vi "HFRR ADV v017 new software.vi"() -> ()   [LabVIEW 2025] (continued)
            n3480 = property on="File Path" class="Path"("Caption.Text"=w4485) -> ()  [unwired: 2 in, 2 out]
            n3481 = property on="SrvM CP" class="Bool (strict)"("Boolean Text.Text"=w4484) -> ()  [unwired: 2 in, 2 out]
            n3482 = local read "S 71"() -> (w4479:string)
            n3483 = local read "S 86"() -> (w4481:string)
            n3484 = local read "S 85"() -> (w4482:string)
            n3485 = local read "S 87"() -> (w4480:string)
            n3486 = local read "S 84"() -> (w4483:string)
            n3487 = local read "S 103"() -> (w4468:string)
            n3488 = local read "S 104"() -> (w4467:string)
            n3489 = property on="ENTER THE NEW PASSWORD" class="Str"("Caption.Text"=w4480) -> ()  [unwired: 2 in, 2 out]
            n3490 = property on="Password" class="Str"("Caption.Text"=w4482) -> ()  [unwired: 2 in, 2 out]
            n3491 = property on="ENTER CURRENT PASSWORD" class="Str"("Caption.Text"=w4481) -> ()  [unwired: 2 in, 2 out]
            n3492 = property on="EDIT" class="Bool (strict)"("Boolean Text.Text"=w4479) -> ()  [unwired: 2 in, 2 out]
            n3493 = property on="SAVE" class="Bool (strict)"("Boolean Text.Text"=w4483) -> ()  [unwired: 2 in, 2 out]
            n3494 = Build Array(w4468, w4467) -> (w4466:string[])
            n3495 = property on="Heater Button" class="Bool (strict)"("Strings [4]"=w4466) -> ()  [unwired: 2 in, 2 out]
            n3496 = property on="CH-HUMIDITY WET" class="DigNum (strict)"("Caption.Size to Text?"=w4469) -> ()  [unwired: 2 in, 2 out]
            n3497 = property on="CH-HUMIDITY DRY" class="DigNum (strict)"("Caption.Size to Text?"=w4469) -> ()  [unwired: 2 in, 2 out]
            n3498 = property on="CH-POWER -" class="DigNum (strict)"("Caption.Size to Text?"=w4469) -> ()  [unwired: 2 in, 2 out]
            n3499 = property on="CH-HEATER" class="DigNum (strict)"("Caption.Size to Text?"=w4469) -> ()  [unwired: 2 in, 2 out]
            n3500 = property on="CH-POWER +" class="DigNum (strict)"("Caption.Size to Text?"=w4469) -> ()  [unwired: 2 in, 2 out]
            n3501 = local read "S 92"() -> (w4478:string)
            n3502 = local read "S 93"() -> (w4477:string)
            n3503 = local read "S 105"() -> (w4464:string)
            n3504 = local read "S 106"() -> (w4463:string)
            n3505 = Build Array(w4478, w4477) -> ()  [unwired: 1 out]
            n3506 = Build Array(w4464, w4463) -> (w4465:string[])
            n3507 = local read "S 95"() -> (w4475:string)
            n3508 = local read "S 94"() -> (w4476:string)
            n3509 = local read "bs"() -> (w4491:string)
            n3510 = local read "as"() -> (w4492:string)
            n3511 = property on="Humidity" class="Bool (strict)"("Strings [4]"=w4465) -> ()  [unwired: 2 in, 2 out]
            n3512 = Concatenate Strings(w4491, "\r", w4492) -> ()  [unwired: 1 out]
            n3513 = property on="STROKE GAIN :" class="DigNum (strict)"("Caption.Text"=w4475) -> ()  [unwired: 2 in, 2 out]
            n3514 = property on="DISPLACEMENT :" class="DigNum (strict)"("Caption.Text"=w4476) -> ()  [unwired: 2 in, 2 out]
            n3515 = property on="Rh After" class="DigNum (strict)"("Caption.Size to Text?"=TRUE ("Caption.Size to Text")) -> ()  [unwired: 2 in, 2 out]
            n3516 = local read "S 48"() -> (w4515:string)
            n3517 = local read "S 50"() -> (w4513:string)
            n3518 = local read "S 51"() -> (w4512:string)
            n3519 = local read "S 49"() -> (w4514:string)
            n3520 = local read "S 52"() -> (w4511:string)
            n3521 = local read "as"() -> (w4496:string)
            n3522 = local read "bs"() -> (w4497:string)
            n3523 = local read "S 56"() -> (w4510:string)
            n3524 = local read "S 57"() -> (w4509:string)
            n3525 = local read "S 58"() -> (w4508:string)
            n3526 = local read "S 59"() -> (w4507:string)
            n3527 = property on="OPEN" class="Bool (strict)"("Boolean Text.Text"=w4511) -> ()  [unwired: 2 in, 2 out]
            n3528 = property on="OPEN 1" class="Bool (strict)"("Boolean Text.Text"=w4515) -> ()  [unwired: 2 in, 2 out]
            n3529 = property on="OPEN 2" class="Bool (strict)"("Boolean Text.Text"=w4514) -> ()  [unwired: 2 in, 2 out]
            n3530 = property on="OPEN 3" class="Bool (strict)"("Boolean Text.Text"=w4513) -> ()  [unwired: 2 in, 2 out]
            n3531 = property on="OPEN 4" class="Bool (strict)"("Boolean Text.Text"=w4512) -> ()  [unwired: 2 in, 2 out]
            n3532 = Concatenate Strings(w4497, "\r", w4496) -> ()  [unwired: 1 out]
            n3533 = local read "S 102"() -> (w4470:string)
            n3534 = property on="КОФ1" class="DigNum (strict)"("Caption.Text"=w4510) -> ()  [unwired: 2 in, 2 out]
            n3535 = local read "S 98"() -> (w4474:string)
            n3536 = local read "S 99"() -> (w4473:string)
            n3537 = local read "S 100"() -> (w4472:string)
            n3538 = local read "S 101"() -> (w4471:string)
            n3539 = property on="КОФ2" class="DigNum (strict)"("Caption.Text"=w4509) -> ()  [unwired: 2 in, 2 out]
            n3540 = property on="КОФ3" class="DigNum (strict)"("Caption.Text"=w4508) -> ()  [unwired: 2 in, 2 out]
            n3541 = property on="КОФ4" class="DigNum (strict)"("Caption.Text"=w4507) -> ()  [unwired: 2 in, 2 out]
            n3542 = local read "bs"() -> (w4495:string)
            n3543 = local read "as"() -> (w4494:string)
            n3544 = property on="CH-POWER +" class="DigNum (strict)"("Caption.Text"=w4474) -> ()  [unwired: 2 in, 2 out]
            n3545 = property on="CH-POWER -" class="DigNum (strict)"("Caption.Text"=w4473) -> ()  [unwired: 2 in, 2 out]
            n3546 = property on="CH-HEATER" class="DigNum (strict)"("Caption.Text"=w4472) -> ()  [unwired: 2 in, 2 out]
            n3547 = property on="CH-HUMIDITY DRY" class="DigNum (strict)"("Caption.Text"=w4471) -> ()  [unwired: 2 in, 2 out]
            n3548 = property on="CH-HUMIDITY WET" class="DigNum (strict)"("Caption.Text"=w4470) -> ()  [unwired: 2 in, 2 out]
            n3549 = local read "S 60"() -> (w4506:string)
            n3550 = local read "S 54"() -> (w4516:string)
            n3551 = Concatenate Strings(w4495, "\r", w4494) -> ()  [unwired: 1 out]
            n3552 = Concatenate Strings(w4516, w4506) -> ()  [unwired: 1 out]
            n3553 = local read "S 77"() -> (→"String 43":string)
            n3554 = local read "S 76"() -> (w4489:string)
            n3555 = local read "S 78"() -> (w4488:string)
            n3556 = local read "S 71"() -> (w4500:string)
            n3557 = local read "S 66"() -> (w4505:string)
            n3558 = local read "S 67"() -> (w4504:string)
            n3559 = local read "S 68"() -> (w4503:string)
            n3560 = local read "S 69"() -> (w4502:string)
            n3561 = local read "S 70"() -> (w4501:string)
            n3562 = property on="AIR TEMP" class="DigNum (strict)"("Caption.Text"=w4488) -> ()  [unwired: 2 in, 2 out]
            n3563 = property on="Set Strk" class="DigNum (strict)"("Caption.Text"=w4489) -> ()  [unwired: 2 in, 2 out]
            n3564 = property on="FRIC. FORCE :" class="DigNum (strict)"("Caption.Text"=w4505) -> ()  [unwired: 2 in, 2 out]
            n3565 = property on="TEMPERATURE :" class="DigNum (strict)"("Caption.Text"=w4504) -> ()  [unwired: 2 in, 2 out]
            n3566 = property on="SPEED OUT:" class="DigNum (strict)"("Caption.Text"=w4503) -> ()  [unwired: 2 in, 2 out]
            n3567 = property on="AIR TEMPERATURE :" class="DigNum (strict)"("Caption.Text"=w4502) -> ()  [unwired: 2 in, 2 out]
            n3568 = property on="HUMIDITY:" class="DigNum (strict)"("Caption.Text"=w4501) -> ()  [unwired: 2 in, 2 out]
            n3569 = property on="EDIT" class="Bool (strict)"("Boolean Text.Text"=w4500) -> ()  [unwired: 2 in, 2 out]
            n3570 = local read "S 79"() -> (w4487:string)
          }
          frame #2 {
          }
        }
        n3571 = local write "Lan flag"(10.0 ("Lan flag")) -> ()
      }
      frame Enabled {
      }
    }
    n3572 = Wait (ms)(milliseconds to wait=u32 2000) -> ()  [unwired: 1 out]
    n3573 = local read "Quit"() -> (w4290:bool)
  }
  n3574 = while {
    shift-right: [w4522] -> _
    shift-left: _ -> [w4523]
    shift-right: [w4520] -> _
    shift-left: T18 {"Read Heave and Surge"="", "Bytes at Heave Port"=0.0, "Heave and Surge COM Port:"="COM9", "Com Port 2"="COM7", "Residual Due"="", "Heave COM Status 2"=TRUE, "Heave COM Status"=TRUE, "Port 2"=TRUE, "Sway PPR"=6400.0, "Surge PPR"=6400.0, "Heave PPR"=6400.0, "Sway Pitch"=2.0, "Surge Pitch"=3.0, "Heave Pitch"=4.0, "Sway Pulses/mm"=320.0, "Surge Pulses/mm"=1600.0, "Heave Pulses/mm"=1600.0, "inner loop"=0.0, "Read Heave and Surge 2"="", "String 36"="", "Write S"=FALSE, "WriteCC1"=[""], "Heave COM Loop"=0, "LastCom"="", "EXIT"=FALSE, "Error Heave"={"status"=TRUE, "code"=-1073807343, "source"=""}} -> [w4519]
    shift-right: [w4517] -> _
    shift-left: _ -> [w4518]
    stop <- w4521 stop-if-true
    n3575 = case shown="\"init\"" w4518 {
      tunnel: w4523 -> [w4537 w4552 w4613 w4615]
      tunnel: [w4532 w4561 w4613 w4615] -> w4522
      tunnel: [_ _ TRUE _] -> w4521
      tunnel: [w4528 w4558 w4611 w4614] -> w4520
      tunnel: w4519 -> [w4534 w4551 w4611 w4614]
      tunnel: [enum16{"init", "MAIN", "Panel Close"}."MAIN" w4545 _ _] -> w4517
      frame "init" {
        n3576 = local read "Com Port 1"() -> (w4524:refnum<visa-resource-name>)
        n3577 = Bundle By Name(cluster=w4534, "Com Port 2"=w4524) -> (w4533:T18)
        n3578 = call "Instrument fgv.vi"("Enum"=T31."INIT", "error in (no error) 2"=w4537, "INPUT"=w4533) -> ("error"=w4535:errorcluster, "output"=w4531:T18)  [unwired: 6 in, 1 out]
        n3579 = case shown="Error" w4535 {
          selector: w4535 -> [w4539 _]
          tunnel: [w4539 w4543] -> w4532
          tunnel: w4531 -> [w4538 w4541]
          tunnel: [w4538 w4540] -> w4529
          frame No Error {
          }
          frame Error {
            n3580 = call "Instrument fgv.vi"("Enum"=T31."ERROR INIT", "INPUT"=w4541) -> ("error"=w4544:errorcluster, "output"=w4540:T18)  [unwired: 7 in, 1 out]
            n3581 = call <vilib>:"Clear Errors.vi"("error in (no error)"=w4544) -> ("error out"=w4543:errorcluster)  [unwired: 5 in, 1 out]
          }
        }
        n3582 = local read "LastCom 2"() -> (w4527:string)
        n3583 = Unbundle By Name(w4529) -> ("Heave COM Status 2"=→"COM Status 2" →"Instrument Status 2":bool, "Error Heave"=→"Error  2":errorcluster)  [unwired: 1 out]
        n3584 = Bundle By Name(cluster=w4529, "LastCom"=w4527) -> (w4528:T18)
      }
      frame "MAIN" {
        n3585 = Unbundle By Name(w4551) -> ("Com Port 2"=w4563:refnum<visa-resource-name>)
        n3586 = local write "Com Port 5"(w4563) -> ()
        n3587 = local read item#-1() -> (w4549)
        n3588 = Bundle By Name(cluster=w4551, "Heave and Surge COM Port:"=w4549) -> (w4550:T18)
        n3589 = Equal?(x=w4563, y=w4549) -> (x = y?=w4562:bool)
        n3590 = case shown="True" w4562 {
          tunnel: [w4567 w4584] -> w4561
          tunnel: w4552 -> [w4568 w4590]
          tunnel: w4550 -> [w4566 w4588]
          tunnel: [w4565 w4583] -> w4558
          frame False {
            n3591 = call <vilib>:"Clear Errors.vi"("error in (no error)"=w4568) -> ("error out"=w4564:errorcluster)  [unwired: 5 in, 1 out]
            n3592 = call "Instrument fgv.vi"("Enum"=T31."ERROR INIT", "error in (no error) 2"=w4564, "INPUT"=w4566) -> ("error"=w4570:errorcluster, "output"=w4565:T18)  [unwired: 6 in, 1 out]
            n3593 = call <vilib>:"Clear Errors.vi"("error in (no error)"=w4570) -> ("error out"=w4567:errorcluster)  [unwired: 5 in, 1 out]
          }
          frame True {
            n3594 = call "Instrument fgv.vi"("Enum"=T31."READ", "error in (no error) 2"=w4590, "INPUT"=w4588) -> ("error"=w4589:errorcluster, "output"=w4580:T18)  [unwired: 6 in, 1 out]
            n3595 = Bundle By Name(cluster=w4580, "String 36"="String 15") -> (w4579:T18)
            n3596 = case shown="True" "Write S 2" {
              selector: "Write S 2" -> [_ w4610]
              tunnel: w4589 -> [w4603 w4609]
              tunnel: [w4603 w4608] -> w4576
              tunnel: w4579 -> [w4602 w4605]
              tunnel: [w4602 w4604] -> w4575
              frame False {
              }
              frame True {
                n3597 = Not(x=w4610) -> (.not. x?=w4606:bool)
                n3598 = local write "Write S 2"(w4606) -> ()
                n3599 = call "Instrument fgv.vi"("Enum"=T31."MANUAL WRITE", "error in (no error) 2"=w4609, "INPUT"=w4605) -> ("error"=w4608:errorcluster, "output"=w4604:T18)  [unwired: 6 in, 1 out]
              }
            }
            n3600 = Array Size(array="WriteHumidity 2") -> (size(s)=w4573:i32)
            n3601 = Greater Than 0?(x=w4573) -> (x > 0?=w4571:bool)
            n3602 = call "Instrument fgv.vi"("Enum"=T31."WRITE", "error in (no error) 2"=w4576, "WriteCC1"="WriteHumidity 2", "INPUT"=w4575) -> ("error"=w4586:errorcluster, "WriteCC1 2"=w4574:string[], "output"=w4585:T18)  [unwired: 5 in]
            n3603 = case shown="Error" w4586 {
              selector: w4586 -> [w4593 w4596]
              tunnel: w4585 -> [w4594 w4601]
              tunnel: [w4594 w4600] -> w4583
              tunnel: [w4593 w4598] -> w4584
              frame No Error {
              }
              frame Error {
                n3604 = call <vilib>:"Clear Errors.vi"("error in (no error)"=w4596) -> ("error out"=w4595:errorcluster)  [unwired: 5 in, 1 out]
                n3605 = call "Instrument fgv.vi"("Enum"=T31."ERROR INIT", "error in (no error) 2"=w4595, "INPUT"=w4601) -> ("error"=w4599:errorcluster, "output"=w4600:T18)  [unwired: 6 in, 1 out]
                n3606 = call <vilib>:"Clear Errors.vi"("error in (no error)"=w4599) -> ("error out"=w4598:errorcluster)  [unwired: 5 in, 1 out]
              }
            }
            n3607 = case shown="True" w4571 {
              tunnel: w4574 -> [_ w4592]
              frame False {
              }
              frame True {
                n3608 = local write "WriteHumidity 2"(w4592) -> ()
              }
            }
            n3609 = Unbundle By Name(w4583) -> ("LastCom"=→"LastCom 2":string, "Read Heave and Surge"=→"Read Humidity 2":string)
          }
        }
        n3610 = Unbundle By Name(w4558) -> ("Heave COM Status 2"=w4560:bool, "Heave COM Status"=w4559:bool, "Error Heave"=w4556:errorcluster, "Bytes at Heave Port"=→"Bytes at Humidity Port  2":dbl)
        n3611 = Unbundle By Name(w4556) -> ("status"=→"Humidity Port 2":bool)
        n3612 = Not(x=w4559) -> (.not. x?=w4553:bool)
        n3613 = local write "Error  2"(w4556) -> ()
        n3614 = Not(x=w4560) -> (.not. x?=w4554:bool)
        n3615 = local write "Instrument Status 2"(w4553) -> ()
        n3616 = local write "COM Status 2"(w4554) -> ()
        n3617 = local read "Quit"() -> (w4546:bool)
        n3618 = Select(t=enum16{"init", "MAIN", "Panel Close"}."Panel Close", s=w4546, f=enum16{"init", "MAIN", "Panel Close"}."MAIN") -> (s? t:f=w4545:enum16{"init", "MAIN", "Panel Close"})
      }
      frame "Panel Close" {
      }
      frame Default {
      }
    }
  }
  n3619 = disable-structure shown="Disabled" {
    frame Disabled {
      n3620 = while {
        tunnel: [w4617] -> _
        i -> [w4617]
        stop <- w4616 continue-if-true
        n3621 = Wait (ms)(milliseconds to wait=u32 50) -> ()  [unwired: 1 out]
        n3622 = stacked-sequence {
          frame #0 {
            # "Controls Text color"
            # "Controls BG color"
            n3623 = property on="FILE" class="Str"("Text.Text Colors:Text Color"="SC  Text") -> ()  [unwired: 2 in, 2 out]
            n3624 = property on="Fuel Discription :" class="Str"("Text.Text Colors:Text Color"="SC  Text") -> ()  [unwired: 2 in, 2 out]
            n3625 = property on="tested by" class="Str"("Text.Text Colors:Text Color"="SC  Text") -> ()  [unwired: 2 in, 2 out]
            n3626 = property on="Remarks :" class="Str"("Text.Text Colors:Text Color"="SC  Text") -> ()  [unwired: 2 in, 2 out]
            n3627 = property class="DigNum (strict)"("Numeric Text.Text Colors:BG Color"="NC BG") -> ()  [unwired: 2 in, 2 out]
            n3628 = property class="DigNum (strict)"("Numeric Text.Text Colors:BG Color"="NC BG") -> ()  [unwired: 2 in, 2 out]
            n3629 = property class="DigNum (strict)"("Numeric Text.Text Colors:BG Color"="NC BG") -> ()  [unwired: 2 in, 2 out]
            n3630 = property class="DigNum (strict)"("Numeric Text.Text Colors:BG Color"="NC BG") -> ()  [unwired: 2 in, 2 out]
            n3631 = property class="DigNum (strict)"("Numeric Text.Text Colors:BG Color"="NC BG") -> ()  [unwired: 2 in, 2 out]
            n3632 = property class="DigNum (strict)"("Numeric Text.Text Colors:BG Color"="NC BG") -> ()  [unwired: 2 in, 2 out]
            n3633 = property class="DigNum (strict)"("Numeric Text.Text Colors:BG Color"="NC BG") -> ()  [unwired: 2 in, 2 out]
            n3634 = property class="DigNum (strict)"("Numeric Text.Text Colors:BG Color"="NC BG") -> ()  [unwired: 2 in, 2 out]
            n3635 = property class="DigNum (strict)"("Numeric Text.Text Colors:BG Color"="NC BG") -> ()  [unwired: 2 in, 2 out]
            n3636 = property class="DigNum (strict)"("Numeric Text.Text Colors:BG Color"="NC BG") -> ()  [unwired: 2 in, 2 out]
            n3637 = property class="DigNum (strict)"("Numeric Text.Text Colors:BG Color"="NC BG") -> ()  [unwired: 2 in, 2 out]
            n3638 = property class="DigNum (strict)"("Numeric Text.Text Colors:BG Color"="NC BG") -> ()  [unwired: 2 in, 2 out]
            n3639 = property on="FILE" class="Str"("Text.Text Colors:BG Color"="SC BG 3") -> ()  [unwired: 2 in, 2 out]
            n3640 = property on="Fuel Discription :" class="Str"("Text.Text Colors:BG Color"="SC BG 3") -> ()  [unwired: 2 in, 2 out]
            n3641 = property on="tested by" class="Str"("Text.Text Colors:BG Color"="SC BG 3") -> ()  [unwired: 2 in, 2 out]
            n3642 = property on="Remarks :" class="Str"("Text.Text Colors:BG Color"="SC BG 3") -> ()  [unwired: 2 in, 2 out]
            n3643 = property class="DigNum (strict)"("Numeric Text.Text Colors:Text Color"="NC Text") -> ()  [unwired: 2 in, 2 out]
            n3644 = property class="DigNum (strict)"("Numeric Text.Text Colors:Text Color"="NC Text") -> ()  [unwired: 2 in, 2 out]
            n3645 = property class="DigNum (strict)"("Numeric Text.Text Colors:Text Color"="NC Text") -> ()  [unwired: 2 in, 2 out]
            n3646 = property class="DigNum (strict)"("Numeric Text.Text Colors:Text Color"="NC Text") -> ()  [unwired: 2 in, 2 out]
            n3647 = property class="DigNum (strict)"("Numeric Text.Text Colors:Text Color"="NC Text") -> ()  [unwired: 2 in, 2 out]
            n3648 = property class="DigNum (strict)"("Numeric Text.Text Colors:Text Color"="NC Text") -> ()  [unwired: 2 in, 2 out]
            n3649 = property class="DigNum (strict)"("Numeric Text.Text Colors:Text Color"="NC Text") -> ()  [unwired: 2 in, 2 out]
            n3650 = property class="DigNum (strict)"("Numeric Text.Text Colors:Text Color"="NC Text") -> ()  [unwired: 2 in, 2 out]
            n3651 = property class="DigNum (strict)"("Numeric Text.Text Colors:Text Color"="NC Text") -> ()  [unwired: 2 in, 2 out]
            n3652 = property class="DigNum (strict)"("Numeric Text.Text Colors:Text Color"="NC Text") -> ()  [unwired: 2 in, 2 out]
            n3653 = property class="DigNum (strict)"("Numeric Text.Text Colors:Text Color"="NC Text") -> ()  [unwired: 2 in, 2 out]
            n3654 = property class="DigNum (strict)"("Numeric Text.Text Colors:Text Color"="NC Text") -> ()  [unwired: 2 in, 2 out]
            n3655 = property class="DigNum (strict)"("Numeric Text.Text Colors:Text Color"="NI Text  2") -> ()  [unwired: 2 in, 2 out]
            n3656 = property class="DigNum (strict)"("Numeric Text.Text Colors:Text Color"="NI Text  2") -> ()  [unwired: 2 in, 2 out]
            n3657 = property class="DigNum (strict)"("Numeric Text.Text Colors:Text Color"="NI Text  2") -> ()  [unwired: 2 in, 2 out]
            n3658 = property class="DigNum (strict)"("Numeric Text.Text Colors:Text Color"="NI Text  2") -> ()  [unwired: 2 in, 2 out]
            n3659 = property class="DigNum (strict)"("Numeric Text.Text Colors:Text Color"="NI Text  2") -> ()  [unwired: 2 in, 2 out]
            n3660 = property class="DigNum (strict)"("Numeric Text.Text Colors:Text Color"="NI Text  2") -> ()  [unwired: 2 in, 2 out]
            n3661 = property class="DigNum (strict)"("Numeric Text.Text Colors:Text Color"="NI Text  2") -> ()  [unwired: 2 in, 2 out]
            n3662 = property class="DigNum (strict)"("Numeric Text.Text Colors:Text Color"="NI Text  2") -> ()  [unwired: 2 in, 2 out]
            n3663 = property class="DigNum (strict)"("Numeric Text.Text Colors:Text Color"="NI Text  2") -> ()  [unwired: 2 in, 2 out]
            n3664 = property class="DigNum (strict)"("Numeric Text.Text Colors:Text Color"="NI Text  2") -> ()  [unwired: 2 in, 2 out]
            n3665 = property class="DigNum (strict)"("Numeric Text.Text Colors:Text Color"="NI Text  2") -> ()  [unwired: 2 in, 2 out]
            n3666 = property class="DigNum (strict)"("Numeric Text.Text Colors:Text Color"="NI Text  2") -> ()  [unwired: 2 in, 2 out]
            n3667 = property class="DigNum (strict)"("Numeric Text.Text Colors:Text Color"="NI Text  2") -> ()  [unwired: 2 in, 2 out]
            n3668 = property class="DigNum (strict)"("Numeric Text.Text Colors:Text Color"="NI Text  2") -> ()  [unwired: 2 in, 2 out]
            n3669 = property class="DigNum (strict)"("Numeric Text.Text Colors:Text Color"="NI Text  2") -> ()  [unwired: 2 in, 2 out]
            n3670 = property on="Coefficient Of Friction" class="XYGraph (strict)"("Plot Area:Colors:FG Color"="GFG  2", "Plot Area:Colors:BG Color"="GBG   2") -> ()  [unwired: 2 in, 2 out]
            n3671 = property on="Humidity ( %RH )" class="XYGraph (strict)"("Plot Area:Colors:FG Color"="GFG  2", "Plot Area:Colors:BG Color"="GBG   2") -> ()  [unwired: 2 in, 2 out]
            n3672 = property on="Air Temperature  ( °C )" class="XYGraph (strict)"("Plot Area:Colors:FG Color"="GFG  2", "Plot Area:Colors:BG Color"="GBG   2") -> ()  [unwired: 2 in, 2 out]
            n3673 = property on="Sample Temperature ( °C )" class="XYGraph (strict)"("Plot Area:Colors:FG Color"="GFG  2", "Plot Area:Colors:BG Color"="GBG   2") -> ()  [unwired: 2 in, 2 out]
            n3674 = property class="DigNum (strict)"("Numeric Text.Text Colors:BG Color"="NI BG 2") -> ()  [unwired: 2 in, 2 out]
            n3675 = property class="DigNum (strict)"("Numeric Text.Text Colors:BG Color"="NI BG 2") -> ()  [unwired: 2 in, 2 out]
            n3676 = property class="DigNum (strict)"("Numeric Text.Text Colors:BG Color"="NI BG 2") -> ()  [unwired: 2 in, 2 out]
            n3677 = property class="DigNum (strict)"("Numeric Text.Text Colors:BG Color"="NI BG 2") -> ()  [unwired: 2 in, 2 out]
            n3678 = property class="DigNum (strict)"("Numeric Text.Text Colors:BG Color"="NI BG 2") -> ()  [unwired: 2 in, 2 out]
            n3679 = property class="DigNum (strict)"("Numeric Text.Text Colors:BG Color"="NI BG 2") -> ()  [unwired: 2 in, 2 out]
            n3680 = property class="DigNum (strict)"("Numeric Text.Text Colors:BG Color"="NI BG 2") -> ()  [unwired: 2 in, 2 out]
            n3681 = property class="DigNum (strict)"("Numeric Text.Text Colors:BG Color"="NI BG 2") -> ()  [unwired: 2 in, 2 out]
            n3682 = property class="DigNum (strict)"("Numeric Text.Text Colors:BG Color"="NI BG 2") -> ()  [unwired: 2 in, 2 out]
            n3683 = property class="DigNum (strict)"("Numeric Text.Text Colors:BG Color"="NI BG 2") -> ()  [unwired: 2 in, 2 out]
            n3684 = property class="DigNum (strict)"("Numeric Text.Text Colors:BG Color"="NI BG 2") -> ()  [unwired: 2 in, 2 out]
            n3685 = property class="DigNum (strict)"("Numeric Text.Text Colors:BG Color"="NI BG 2") -> ()  [unwired: 2 in, 2 out]
            n3686 = property class="DigNum (strict)"("Numeric Text.Text Colors:BG Color"="NI BG 2") -> ()  [unwired: 2 in, 2 out]
            n3687 = property class="DigNum (strict)"("Numeric Text.Text Colors:BG Color"="NI BG 2") -> ()  [unwired: 2 in, 2 out]
            n3688 = property class="DigNum (strict)"("Numeric Text.Text Colors:BG Color"="NI BG 2") -> ()  [unwired: 2 in, 2 out]
            n3689 = property class="Bool"("Colors [4]"="Boolean BC T & BG") -> ()  [unwired: 2 in, 2 out]
            n3690 = property on="Save & Continue" class="Bool (strict)"("Colors [4]"="Boolean BC T & BG") -> ()  [unwired: 2 in, 2 out]
            n3691 = property on="Heater Button" class="Bool (strict)"("Colors [4]"="Boolean BC T & BG") -> ()  [unwired: 2 in, 2 out]
            n3692 = property class="Bool"("Colors [4]"="Boolean BC T & BG") -> ()  [unwired: 2 in, 2 out]
            n3693 = property on="Humidity" class="Bool (strict)"("Colors [4]"="Boolean BC T & BG") -> ()  [unwired: 2 in, 2 out]
            n3694 = property class="Bool (strict)"("Colors [4]"="Boolean BC T & BG") -> ()  [unwired: 2 in, 2 out]
            n3695 = property on="RUN" class="Bool (strict)"("Colors [4]"="Boolean BC T & BG") -> ()  [unwired: 2 in, 2 out]
            n3696 = property on="trip1 8" class="Bool (strict)"("Colors [4]"="Boolean BC T & BG") -> ()  [unwired: 2 in, 2 out]
            n3697 = property class="Bool"("Colors [4]"="Boolean BC T & BG") -> ()  [unwired: 2 in, 2 out]
            n3698 = property class="Bool (strict)"("Colors [4]"="Boolean BC T & BG") -> ()  [unwired: 2 in, 2 out]
            n3699 = property on="OPEN 1" class="Bool (strict)"("Colors [4]"="Boolean BC T & BG 2") -> ()  [unwired: 2 in, 2 out]
            n3700 = property on="OPEN 2" class="Bool (strict)"("Colors [4]"="Boolean BC T & BG 2") -> ()  [unwired: 2 in, 2 out]
            n3701 = property on="OPEN 3" class="Bool (strict)"("Colors [4]"="Boolean BC T & BG 2") -> ()  [unwired: 2 in, 2 out]
            n3702 = property on="OPEN 4" class="Bool (strict)"("Colors [4]"="Boolean BC T & BG 2") -> ()  [unwired: 2 in, 2 out]
            n3703 = property on="OPEN" class="Bool (strict)"("Colors [4]"="Boolean BC T & BG 2") -> ()  [unwired: 2 in, 2 out]
            n3704 = property on="rstv2" class="Bool"("Colors [4]"="Boolean BC T & BG 2") -> ()  [unwired: 2 in, 2 out]
            n3705 = property on="RST CP" class="Bool"("Colors [4]"="Boolean BC T & BG 2") -> ()  [unwired: 2 in, 2 out]
            n3706 = property on="RSTV1 3" class="Bool"("Colors [4]"="Boolean BC T & BG 2") -> ()  [unwired: 2 in, 2 out]
            n3707 = property on="RSTV1 2" class="Bool"("Colors [4]"="Boolean BC T & BG 2") -> ()  [unwired: 2 in, 2 out]
          }
          frame #1 {
          }
        }
        n3708 = local read "Quit"() -> (w4616:bool)
      }
    }
    frame Enabled {
    }
  }
  n3709 = while {
    shift-right: [w4634] -> _
    shift-left: _ -> [w4635]
    shift-right: [w4632] -> _
    shift-left: T18 {"Read Heave and Surge"="", "Bytes at Heave Port"=0.0, "Heave and Surge COM Port:"="COM9", "Com Port 2"="COM7", "Residual Due"="", "Heave COM Status 2"=TRUE, "Heave COM Status"=TRUE, "Port 2"=TRUE, "Sway PPR"=6400.0, "Surge PPR"=6400.0, "Heave PPR"=6400.0, "Sway Pitch"=2.0, "Surge Pitch"=3.0, "Heave Pitch"=4.0, "Sway Pulses/mm"=320.0, "Surge Pulses/mm"=1600.0, "Heave Pulses/mm"=1600.0, "inner loop"=0.0, "Read Heave and Surge 2"="", "String 36"="", "Write S"=FALSE, "WriteCC1"=[""], "Heave COM Loop"=0, "LastCom"="", "EXIT"=FALSE, "Error Heave"={"status"=TRUE, "code"=-1073807343, "source"=""}} -> [w4631]
    shift-right: [w4629] -> _
    shift-left: enum16{"init", "MAIN", "Panel Close"}."init" -> [w4630]
    stop <- w4633 stop-if-true
    n3710 = case shown="\"init\"" w4630 {
      tunnel: w4635 -> [w4649 w4664 w4725 w4727]
      tunnel: [w4643 w4673 w4725 w4727] -> w4634
      tunnel: [_ _ TRUE _] -> w4633
      tunnel: [w4639 w4670 w4723 w4726] -> w4632
      tunnel: w4631 -> [w4646 w4663 w4723 w4726]
      tunnel: [enum16{"init", "MAIN", "Panel Close"}."MAIN" w4657 _ _] -> w4629
      frame "init" {
        n3711 = Bundle By Name(cluster=w4646, "Heave and Surge COM Port:"="C3 :") -> (w4645:T18)
        n3712 = call "Instrument fgv.vi"("Enum"=T31."INIT", "error in (no error) 2"=w4649, "INPUT"=w4645) -> ("error"=w4647:errorcluster, "output"=w4642:T18)  [unwired: 6 in, 1 out]
        n3713 = case shown="Error" w4647 {
          selector: w4647 -> [w4651 _]
          tunnel: [w4651 w4655] -> w4643
          tunnel: w4642 -> [w4650 w4653]
          tunnel: [w4650 w4652] -> w4640
          frame No Error {
          }
          frame Error {
            n3714 = call "Instrument fgv.vi"("Enum"=T31."ERROR INIT", "INPUT"=w4653) -> ("error"=w4656:errorcluster, "output"=w4652:T18)  [unwired: 7 in, 1 out]
            n3715 = call <vilib>:"Clear Errors.vi"("error in (no error)"=w4656) -> ("error out"=w4655:errorcluster)  [unwired: 5 in, 1 out]
          }
        }
        n3716 = local read "LastCom"() -> (w4638:string)
        n3717 = Unbundle By Name(w4640) -> ("Heave COM Status 2"=→"COM Status" →"Instrument Status":bool, "Error Heave"=→"Error":errorcluster)  [unwired: 1 out]
        n3718 = Bundle By Name(cluster=w4640, "LastCom"=w4638) -> (w4639:T18)
      }
      frame "MAIN" {
        n3719 = Unbundle By Name(w4663) -> ("Com Port 2"=w4675:refnum<visa-resource-name>)
        n3720 = local write "Com Port 4"(w4675) -> ()
        n3721 = local read "C3 :"() -> (w4661:refnum<visa-resource-name>)
        n3722 = Bundle By Name(cluster=w4663, "Heave and Surge COM Port:"=w4661) -> (w4662:T18)
        n3723 = Equal?(x=w4675, y=w4661) -> (x = y?=w4674:bool)
        n3724 = case shown="True" w4674 {
          tunnel: [w4679 w4696] -> w4673
          tunnel: w4664 -> [w4680 w4702]
          tunnel: w4662 -> [w4678 w4700]
          tunnel: [w4677 w4695] -> w4670
          frame False {
            n3725 = call <vilib>:"Clear Errors.vi"("error in (no error)"=w4680) -> ("error out"=w4676:errorcluster)  [unwired: 5 in, 1 out]
            n3726 = call "Instrument fgv.vi"("Enum"=T31."ERROR INIT", "error in (no error) 2"=w4676, "INPUT"=w4678) -> ("error"=w4682:errorcluster, "output"=w4677:T18)  [unwired: 6 in, 1 out]
            n3727 = call <vilib>:"Clear Errors.vi"("error in (no error)"=w4682) -> ("error out"=w4679:errorcluster)  [unwired: 5 in, 1 out]
          }
          frame True {
            n3728 = call "Instrument fgv.vi"("Enum"=T31."READ", "error in (no error) 2"=w4702, "INPUT"=w4700) -> ("error"=w4701:errorcluster, "output"=w4692:T18)  [unwired: 6 in, 1 out]
            n3729 = Bundle By Name(cluster=w4692, "String 36"="String 11") -> (w4691:T18)
            n3730 = case shown="True" "Write S" {
              selector: "Write S" -> [_ w4722]
              tunnel: w4701 -> [w4715 w4721]
              tunnel: [w4715 w4720] -> w4688
              tunnel: w4691 -> [w4714 w4717]
              tunnel: [w4714 w4716] -> w4687
              frame False {
              }
              frame True {
                n3731 = Not(x=w4722) -> (.not. x?=w4718:bool)
                n3732 = local write "Write S"(w4718) -> ()
                n3733 = call "Instrument fgv.vi"("Enum"=T31."MANUAL WRITE", "error in (no error) 2"=w4721, "INPUT"=w4717) -> ("error"=w4720:errorcluster, "output"=w4716:T18)  [unwired: 6 in, 1 out]
              }
            }
            n3734 = Array Size(array="WriteHumidity") -> (size(s)=w4685:i32)
            n3735 = Greater Than 0?(x=w4685) -> (x > 0?=w4683:bool)
            n3736 = call "Instrument fgv.vi"("Enum"=T31."WRITE", "error in (no error) 2"=w4688, "WriteCC1"="WriteHumidity", "INPUT"=w4687) -> ("error"=w4698:errorcluster, "WriteCC1 2"=w4686:string[], "output"=w4697:T18)  [unwired: 5 in]
            n3737 = case shown="True" w4683 {
              tunnel: w4686 -> [_ w4704]
              frame False {
              }
              frame True {
                n3738 = local write "WriteHumidity"(w4704) -> ()
              }
            }
            n3739 = case shown="Error" w4698 {
              selector: w4698 -> [w4705 w4708]
              tunnel: w4697 -> [w4706 w4713]
              tunnel: [w4706 w4712] -> w4695
              tunnel: [w4705 w4710] -> w4696
              frame No Error {
              }
              frame Error {
                n3740 = call <vilib>:"Clear Errors.vi"("error in (no error)"=w4708) -> ("error out"=w4707:errorcluster)  [unwired: 5 in, 1 out]
                n3741 = call "Instrument fgv.vi"("Enum"=T31."ERROR INIT", "error in (no error) 2"=w4707, "INPUT"=w4713) -> ("error"=w4711:errorcluster, "output"=w4712:T18)  [unwired: 6 in, 1 out]
                n3742 = call <vilib>:"Clear Errors.vi"("error in (no error)"=w4711) -> ("error out"=w4710:errorcluster)  [unwired: 5 in, 1 out]
              }
            }
            n3743 = Unbundle By Name(w4695) -> ("LastCom"=→"LastCom":string, "Read Heave and Surge"=→"Read Humidity":string)
          }
        }
        n3744 = Unbundle By Name(w4670) -> ("Heave COM Status 2"=w4672:bool, "Heave COM Status"=w4671:bool, "Error Heave"=w4668:errorcluster, "Bytes at Heave Port"=→"Bytes at Humidity Port":dbl)
        n3745 = Unbundle By Name(w4668) -> ("status"=→"Humidity Port":bool)
        n3746 = Not(x=w4671) -> (.not. x?=w4665:bool)
        n3747 = local write "Error"(w4668) -> ()
        n3748 = Not(x=w4672) -> (.not. x?=w4666:bool)
        n3749 = local write "Instrument Status"(w4665) -> ()
        n3750 = local write "COM Status"(w4666) -> ()
        n3751 = local read "Quit"() -> (w4658:bool)
        n3752 = Select(t=enum16{"init", "MAIN", "Panel Close"}."Panel Close", s=w4658, f=enum16{"init", "MAIN", "Panel Close"}."MAIN") -> (s? t:f=w4657:enum16{"init", "MAIN", "Panel Close"})
      }
      frame "Panel Close" {
      }
      frame Default {
      }
    }
  }
  n3753 = while {
    stop <- w4753 stop-if-true
    n3754 = local read "Read Humidity"() -> (w4734:string)
    n3755 = call <vilib>:"High Resolution Polling Wait.vi"("seconds to wait"=0.1) -> ()  [unwired: 10 in, 1 out]
    n3756 = Spreadsheet String To Array(delimiter (Tab)=",", format string="", spreadsheet string=w4734, array type (2D Dbl)=string[] []) -> (array=w4748:string[])
    n3757 = for {
      tunnel: w4748 -> [w4758] mode=indexing
      tunnel: string[] ["STATE;", "SET;", "RH;", "T;", "AMB_RH;", "AMB_T;", "PUMP;", "FAN_IN;", "FAN_OUT;", "DEHUM;", "CURRENT;", "STALL;"] -> [w4757] mode=indexing
      tunnel: [w4756] -> w4747 mode=indexing
      n3758 = Match Pattern(string=w4758, regular expression=w4757) -> (after substring=w4756:string)  [unwired: 1 in, 3 out]
    }
    n3759 = Index Array(array=w4747) -> (element #1=→"STATE :":string, element #2=→"SET :":string, element #3=w4736:string, element #4=→"T :":string, element #5=w4733:string, element #6=→"AMB_T :":string, element #7=→"PUMP :":string, element #8=→"FAN_IN :":string, element #9=→"FAN_OUT :":string, element #10=→"DEHUM :":string, element #11=→"CURRENT :":string, element #12=→"STALL :":string)  [unwired: 12 in]
    "RH :" <- w4736
    "AMB_RH :" <- w4733
    n3760 = Fract/Exp String To Number(string=w4736) -> (number=w4728:dbl)  [unwired: 3 in, 1 out]
    n3761 = Fract/Exp String To Number(string=w4733) -> (number=w4732:dbl)  [unwired: 3 in, 1 out]
    n3762 = local write "Ambient Humidity :"(w4732) -> ()
    n3763 = Equal?(x=w4728, y=0.0) -> (x = y?=w4730:bool)
    n3764 = case shown="True" w4730 {
      tunnel: [w4754 w4755] -> w4729
      tunnel: w4728 -> [w4754 _]
      frame False {
        (unwired) 0.0
        "Humidity temp" <- w4754
      }
      frame True {
        n3765 = local read "Humidity temp"() -> (w4755:dbl)
      }
    }
    "RH Numeric:" <- w4729
    n3766 = local read "Quit"() -> (w4753:bool)
  }
  n3767 = disable-structure shown="Disabled" {
    frame Disabled {
      n3768 = while {
        tunnel: [w4992] -> _
        i -> [w4992]
        stop <- w4989 stop-if-true
        n3769 = local read "powstat"() -> (w4990:bool)
        n3770 = case shown="True" w4990 {
          frame False {
          }
          frame True {
            n3771 = local read "RUN"() -> (w4993:bool)
            n3772 = case shown="True" w4993 {
              frame False {
                w5023 = 65.0 ("y")
                n3773 = local read "Set Hz"() -> (w5051:dbl)
                n3774 = local read "NORMAL LOAD"() -> (w5052:dbl)
                n3775 = Multiply(x=w5051, y=60.0) -> (x*y=w5058:dbl)
                n3776 = Multiply(x=1.2 ("y"), y=0.949) -> (x*y=w5027:dbl)
                n3777 = Multiply(x=1.2 ("y"), y=0.8166) -> (x*y=w5031:dbl)
                n3778 = Multiply(x=1.2 ("y"), y=0.851) -> (x*y=w5026:dbl)
                n3779 = local read "FF 2"() -> (w5050:dbl)
                n3780 = Absolute Value(x=w5058) -> (abs(x)=w5056:dbl)
                n3781 = case shown="13.." w5050 {
                  tunnel: [1 2 3] -> w5048
                  frame 0..10, Default {
                    # "Normal"
                  }
                  frame 11, 12 {
                  }
                  frame 13.. {
                  }
                }
                "FF STATE" <- w5048
                n3782 = local read "TEMP"() -> (w5011:dbl)
                n3783 = local read item#-1() -> (w5025)
                n3784 = Less?(x=w5025, y=w5031) -> (x < y?=w5028:bool)
                n3785 = In Range and Coerce(upper limit=w5027, x=w5025, lower limit=w5026) -> (In Range?=w5029:bool)  [unwired: 1 out]
                n3786 = case shown="3601.." w5056 {
                  tunnel: [1 2 3] -> w5054
                  frame 0..3000, Default {
                    # "Normal"
                  }
                  frame 3001..3600 {
                  }
                  frame 3601.. {
                  }
                }
                n3787 = case shown="11.." w5052 {
                  tunnel: [1 3] -> w5053
                  frame 1..10, Default {
                  }
                  frame 11.. {
                  }
                }
                "NL STATE" <- w5053
                n3788 = Multiply(x=1.2 ("y"), y=0.95) -> (x*y=w5041:dbl)
                n3789 = Multiply(x=w5023, y=0.954) -> (x*y=w5015:dbl)
                n3790 = Or(x=w5028, y=w5029) -> (x .or. y?=w5030:bool)
                n3791 = Greater Or Equal?(x=w5025, y=w5041) -> (x >= y?=w5038:bool)
                n3792 = Multiply(x=w5023, y=0.99) -> (x*y=w5012:dbl)
                n3793 = Greater Or Equal?(x=w5011, y=w5012) -> (x >= y?=w5017:bool)
                n3794 = Greater Or Equal?(x=w5011, y=w5015) -> (x >= y?=w5014:bool)
                n3795 = case shown="0, 1, Default" w5025 {
                  tunnel: [1 3] -> w5042
                  frame 0, 1, Default {
                  }
                  frame 2.. {
                  }
                }
                n3796 = case shown="True" w5038 {
                  tunnel: [1 3] -> w5043
                  frame False {
                  }
                  frame True {
                  }
                }
                n3797 = case shown="True" w5030 {
                  tunnel: [1 2] -> w5044
                  frame False {
                  }
                  frame True {
                  }
                }
                n3798 = case shown="..0" w5011 {
                  tunnel: [2 3 3 1] -> w5018
                  frame 61, 62 {
                  }
                  frame 63.. {
                  }
                  frame ..0 {
                  }
                  frame 10..60, Default {
                  }
                }
                n3799 = case shown="True" w5017 {
                  tunnel: [1 3] -> w5019
                  frame False {
                  }
                  frame True {
                  }
                }
                n3800 = Number To Decimal String(number=w5054) -> (decimal integer string=w5055:string)  [unwired: 1 in]
                n3801 = case shown="True" w5014 {
                  tunnel: [1 2] -> w5020
                  frame False {
                  }
                  frame True {
                  }
                }
                n3802 = Number To Decimal String(number=1) -> (decimal integer string=→"Air temp":string)  [unwired: 1 in]
                n3803 = Number To Decimal String(number=w5048) -> (decimal integer string=→"ff_st":string)  [unwired: 1 in]
                n3804 = local write "sp_st"(w5055) -> ()
                n3805 = Number To Decimal String(number=w5053) -> (decimal integer string=→"nl_st":string)  [unwired: 1 in]
                n3806 = Build Array(w5018, w5019, w5020) -> (w5021:i32[])
                n3807 = Build Array(w5042, w5043, w5044) -> (w5045:i32[])
                n3808 = Array Max & Min(array=w5021) -> (max value=w5022:i32)  [unwired: 3 out]
                n3809 = Array Max & Min(array=w5045) -> (max value=w5046:i32)  [unwired: 3 out]
                n3810 = Number To Decimal String(number=w5022) -> (decimal integer string=w5010:string)  [unwired: 1 in]
                n3811 = Number To Decimal String(number=w5046) -> (decimal integer string=→"Stroke Ln 2":string)  [unwired: 1 in]
                n3812 = local write "temp_st"(w5010) -> ()
              }
              frame True {
                w5108 = 65.0 ("y")
                # "Healthy -1\nWarning -2\nError -3"
                n3813 = local read "TEMP"() -> (w5119:dbl)
                n3814 = local read "NORMAL LOAD"() -> (w5123:dbl)
                n3815 = local read "Set Hz"() -> (w5121:dbl)
                n3816 = Multiply(x=1.2 ("y"), y=0.949) -> (x*y=w5103:dbl)
                n3817 = Multiply(x=1.2 ("y"), y=0.8166) -> (x*y=w5099:dbl)
                n3818 = Multiply(x=1.2 ("y"), y=0.851) -> (x*y=w5104:dbl)
                n3819 = Multiply(x=w5108, y=0.954) -> (x*y=w5115:dbl)
                n3820 = Multiply(x=w5108, y=0.99) -> (x*y=w5118:dbl)
                n3821 = Greater Or Equal?(x=w5119, y=w5118) -> (x >= y?=w5113:bool)
                n3822 = Multiply(x=w5121, y=60.0) -> (x*y=w5127:dbl)
                n3823 = Greater Or Equal?(x=w5119, y=w5115) -> (x >= y?=w5116:bool)
                n3824 = local read "FF 2"() -> (w5122:dbl)
                n3825 = local read item#-1() -> (w5105)
                n3826 = Less?(x=w5105, y=w5099) -> (x < y?=w5102:bool)
                n3827 = In Range and Coerce(upper limit=w5103, x=w5105, lower limit=w5104) -> (In Range?=w5101:bool)  [unwired: 1 out]
                n3828 = Absolute Value(x=w5127) -> (abs(x)=w5125:dbl)
                n3829 = case shown="63.." w5119 {
                  tunnel: [2 3 3 1] -> w5112
                  frame 61, 62 {
                  }
                  frame 63.. {
                  }
                  frame ..0 {
                  }
                  frame 10..60, Default {
                  }
                }
                n3830 = case shown="True" w5113 {
                  tunnel: [1 3] -> w5111
                  frame False {
                  }
                  frame True {
                  }
                }
                n3831 = case shown="True" w5116 {
                  tunnel: [1 2] -> w5110
                  frame False {
                  }
                  frame True {
                  }
                }
                n3832 = Multiply(x=1.2 ("y"), y=0.95) -> (x*y=w5089:dbl)
                n3833 = case shown="1..10, Default" w5123 {
                  tunnel: [1 3] -> w5130
                  frame 1..10, Default {
                  }
                  frame 11.. {
                  }
                }
                n3834 = case shown="0..10, Default" w5122 {
                  tunnel: [1 2 3] -> w5129
                  frame 0..10, Default {
                  }
                  frame 11, 12 {
                  }
                  frame 13.. {
                  }
                }
                n3835 = case shown="3601.." w5125 {
                  tunnel: [1 2 3] -> w5124
                  frame 0..3000, Default {
                    # "Normal"
                  }
                  frame 3001..3600 {
                  }
                  frame 3601.. {
                  }
                }
                n3836 = Or(x=w5102, y=w5101) -> (x .or. y?=w5100:bool)
                n3837 = Greater Or Equal?(x=w5105, y=w5089) -> (x >= y?=w5092:bool)
                n3838 = case shown="0, 1, Default" w5105 {
                  tunnel: [1 3] -> w5088
                  frame 0, 1, Default {
                  }
                  frame 2.. {
                  }
                }
                n3839 = case shown="True" w5092 {
                  tunnel: [1 3] -> w5087
                  frame False {
                  }
                  frame True {
                  }
                }
                n3840 = case shown="True" w5100 {
                  tunnel: [1 2] -> w5086
                  frame False {
                  }
                  frame True {
                  }
                }
                n3841 = Build Array(w5112, w5111, w5110) -> (w5109:i32[])
                n3842 = Number To Decimal String(number=w5124) -> (decimal integer string=→"sp_st":string)  [unwired: 1 in]
                n3843 = Array Max & Min(array=w5109) -> (max value=w5106:i32)  [unwired: 3 out]
                "TEMP STATE" <- w5106
                n3844 = Number To Decimal String(number=w5130) -> (decimal integer string=w5133:string)  [unwired: 1 in]
                n3845 = Number To Decimal String(number=w5129) -> (decimal integer string=w5131:string)  [unwired: 1 in]
                n3846 = Number To Decimal String(number=w5106) -> (decimal integer string=→"temp_st":string)  [unwired: 1 in]
                n3847 = Build Array(w5088, w5087, w5086) -> (w5085:i32[])
                n3848 = local write "nl_st"(w5133) -> ()
                n3849 = local write "ff_st"(w5131) -> ()
                n3850 = Number To Decimal String(number=1) -> (decimal integer string=w5128:string)  [unwired: 1 in]
                n3851 = Array Max & Min(array=w5085) -> (max value=w5084:i32)  [unwired: 3 out]
                n3852 = local write "Air temp"(w5128) -> ()
                n3853 = Number To Decimal String(number=w5084) -> (decimal integer string=w5083:string)  [unwired: 1 in]
                n3854 = local write "Stroke Ln 2"(w5083) -> ()
              }
            }
            n3855 = local read "Stroke Ln 2"() -> (w4995:string)
            n3856 = local read "nl_st"() -> (w5001:string)
            n3857 = local read "ff_st"() -> (w4998:string)
            n3858 = local read "sp_st"() -> (w4999:string)
            n3859 = local read "temp_st"() -> (w5000:string)
            n3860 = local read "Air temp"() -> (w4994:string)
            n3861 = Replace Array Subset(array="in", new element #1=w5001, index #1=1 ("index"), new element #2=w4998, index #2=2 ("index"), new element #3=w5000, index #3=3 ("index"), new element #4=w4999, index #4=4 ("index"), new element #5=w4995, index #5=5 ("index"), new element #6=w4994, index #6=6 ("index"), new element #7="Sensor State" ("new element/subarray"), index #7=0 ("index")) -> (→"out":string[])
          }
        }
        n3862 = Wait (ms)(milliseconds to wait=u32 10) -> ()  [unwired: 1 out]
        n3863 = local read "Quit"() -> (w4989:bool)
      }
      n3864 = while {
        stop <- w4964 stop-if-true
        n3865 = local read "run replace"() -> (w4966:bool)
        n3866 = Wait (ms)(milliseconds to wait=u32 100) -> ()  [unwired: 1 out]
        n3867 = Equal?(x="FLAG 2", y=0.0) -> (x = y?=w4967:bool)
        n3868 = case shown="True" w4967 {
          frame False {
          }
          frame True {
            n3869 = local write "FLAG 2"(100.0 ("FLAG 2")) -> ()
            n3870 = call <vilib>:"Read Characters From File.vi"("file path (dialog if empty)"=path "C:/LAB-IQ-NXT/WO 2449 TT.sig", "convert eol? (no:F)"=FALSE ("append to file? (new file:F)")) -> ("character string"=w4970:string)  [unwired: 4 in, 3 out]
            n3871 = call <vilib>:"Read Characters From File.vi"("file path (dialog if empty)"=path "C:/LAB-IQ-NXT/WO 2449 TRH.sig", "convert eol? (no:F)"=FALSE ("append to file? (new file:F)")) -> ("character string"=w4971:string)  [unwired: 4 in, 3 out]
            n3872 = Decimal String To Number(string=w4970) -> (number=w4972:i32)  [unwired: 2 in, 1 out]
            n3873 = local write "Total No. of Tests"(w4972) -> ()
            n3874 = Decimal String To Number(string=w4971) -> (number=w4975:i32)  [unwired: 2 in, 1 out]
            n3875 = local write "SEN.RUN HRS"(w4975) -> ()
          }
        }
        n3876 = case shown="True" w4966 {
          frame False {
          }
          frame True {
            n3877 = Equal?(x="FLAG 4", y=0.0) -> (x = y?=w4979:bool)
            n3878 = case shown="False" w4979 {
              frame False {
                n3879 = Get Date/Time In Seconds() -> (seconds since 1Jan1904=w4985:timestamp)
                n3880 = local read "START 3"() -> (w4983:dbl)
                n3881 = To Double Precision Float(number=w4985) -> (double precision float=w4984:dbl)
                n3882 = Subtract(x=w4984, y=w4983) -> (x-y=→"SENSOR TIME":dbl)
              }
              frame True {
                n3883 = Get Date/Time In Seconds() -> (seconds since 1Jan1904=w4987:timestamp)
                n3884 = local write "FLAG 4"(100.0 ("FLAG")) -> ()
                n3885 = To Double Precision Float(number=w4987) -> (double precision float=→"START 3":dbl)
              }
            }
          }
        }
        n3886 = local read "Quit"() -> (w4964:bool)
      }
      n3887 = while {
        shift-right: [w4764] -> _
        shift-left: _ -> [w4765]
        tunnel: [w4760] -> _
        i -> [w4760]
        stop <- w4759 stop-if-true
        n3888 = Wait (ms)(milliseconds to wait=u32 50 ("Refresh Rate (ms)")) -> ()  [unwired: 1 out]
        n3889 = local read "Json End Flg"() -> (w4761:bool)
        n3890 = Not(x="Upld AR 2") -> ()  [unwired: 1 out]
        n3891 = local read "Upld AR 2"() -> (w4762:bool)
        n3892 = call "Elapsed Time9"("Time Target (s)"="Sen.Upload Rate (s)", "Reset"=FALSE, "Auto Reset"=TRUE) -> ("Time has Elapsed"=w4771:bool)  [unwired: 9 in, 7 out]
        n3893 = Or(x=w4771, y=w4761) -> (x .or. y?=w4767:bool)
        n3894 = case shown="True" w4767 {
          frame False {
          }
          frame True {
            w4863 = "\"SensorName\":\"" ("string")
            w4833 = " \"},{"
            w4858 = "\",\"SensorState\":\""
            w4860 = "\",\"SensorModelNumber\":\"" ("string")
            w4859 = "\",\"SensorRuntimeHours\":\"" ("string")
            n3895 = local read "model num"() -> (w4857:string[])
            n3896 = local read "Sensor name"() -> (w4876:string[])
            n3897 = local read "run"() -> (w4847:string[])
            n3898 = local read "SENSOR TIME"() -> (w4803:dbl)
            n3899 = local read "out"() -> (w4796:string[])
            n3900 = local read "Total No. of Tests"() -> (w4801:dbl)
            n3901 = Select(t=60.0, s="Run test 3", f=3600.0) -> (s? t:f=w4811:dbl)
            n3902 = Index Array(array=w4857, index #1=1 ("index")) -> (element #1=w4856:string, element #2=w4855:string, element #3=w4854:string, element #4=w4853:string, element #5=w4852:string, element #6=w4851:string)  [unwired: 5 in]
            n3903 = Index Array(array=w4847, index #1=1 ("index")) -> (element #1=w4846:string, element #2=w4845:string, element #3=w4844:string, element #4=w4843:string, element #5=w4842:string, element #6=w4841:string)  [unwired: 5 in]
            n3904 = Index Array(array=w4876, index #1=1 ("index")) -> (element #1=w4875:string, element #2=w4874:string, element #3=w4873:string, element #4=w4872:string, element #5=w4862:string, element #6=w4861:string)  [unwired: 5 in]
            n3905 = Index Array(array=w4796, index #1=1 ("index")) -> (element #1=w4828:string, element #2=w4827:string, element #3=w4826:string, element #4=w4825:string, element #5=w4824:string, element #6=w4823:string)  [unwired: 5 in]
            n3906 = local read "SEN.RUN HRS"() -> (w4799:dbl)
            n3907 = Divide(x=w4803, y=w4811) -> (x/y=w4810:dbl)
            n3908 = Increment(x=w4810) -> (x+1=w4806:dbl)
            n3909 = Number To Decimal String(number=w4806) -> (decimal integer string=→"run hrs":string)  [unwired: 1 in]
            n3910 = Divide(x=w4799, y=3600.0 ("f")) -> (x/y=w4794:dbl)
            n3911 = Round To Nearest(number=w4794) -> (nearest integer value=w4792:dbl)
            n3912 = Number To Decimal String(number=w4792) -> (decimal integer string=w4793:string)  [unwired: 1 in]
            n3913 = Number To Decimal String(number=w4801) -> (decimal integer string=w4802:string)  [unwired: 1 in]
            n3914 = local read "Model No"() -> (w4807:string)
            n3915 = local read "UUID"() -> (w4902:string)
            n3916 = local read "Serial No"() -> (w4906:string)
            n3917 = local read "Secret Key"() -> (w4907:string)
            n3918 = Concatenate Strings("\",\"MachineSerialNumber\":\"" ("string"), w4906) -> (w4910:string)
            n3919 = Concatenate Strings("\",\"ModelNumber\":\"" ("string"), w4807) -> (w4808:string)
            n3920 = Concatenate Strings("\",\"MachineRuntimeHours\":\"" ("string"), w4793) -> (w4911:string)
            n3921 = Concatenate Strings("\",\"MachineRuntimeCycles\":\"", w4802) -> (w4904:string)
            n3922 = Concatenate Strings(w4860, w4856) -> (w4890:string)
            n3923 = Concatenate Strings(w4859, w4846) -> (w4891:string)
            n3924 = Concatenate Strings(w4858, w4828) -> (w4889:string)
            n3925 = Concatenate Strings(w4910, w4808, w4911, w4904) -> (w4913:string)
            n3926 = Concatenate Strings(w4860, w4855) -> (w4887:string)
            n3927 = Concatenate Strings(w4859, w4845) -> (w4886:string)
            n3928 = Concatenate Strings(w4858, w4827) -> (w4888:string)
            n3929 = Concatenate Strings(w4860, w4854) -> (w4882:string)
            n3930 = Concatenate Strings(w4859, w4844) -> (w4883:string)
            n3931 = Concatenate Strings(w4858, w4826) -> (w4881:string)
            n3932 = Concatenate Strings(w4860, w4853) -> (w4879:string)
            n3933 = Concatenate Strings(w4859, w4843) -> (w4878:string)
            n3934 = Concatenate Strings(w4858, w4825) -> (w4880:string)
            n3935 = Concatenate Strings(w4890, w4891, w4889) -> (w4892:string)
            n3936 = Concatenate Strings(w4860, w4852) -> (w4869:string)
            n3937 = Concatenate Strings(w4859, w4842) -> (w4870:string)
            n3938 = Concatenate Strings(w4860, w4851) -> (w4866:string)
            n3939 = Concatenate Strings(w4859, w4841) -> (w4865:string)
            n3940 = Concatenate Strings(w4858, w4824) -> (w4868:string)
            n3941 = Concatenate Strings(w4858, w4823) -> (w4867:string)
            n3942 = Concatenate Strings("{\"SecretKey\":\"", w4907, w4913, "\",\"UUID\" : \"", w4902, "\",\"SensorInformation\":", "[{" ("string")) -> (w4840:string)
            n3943 = Concatenate Strings(w4887, w4886, w4888) -> (w4885:string)
            n3944 = Concatenate Strings(w4882, w4883, w4881) -> (w4884:string)
            n3945 = Concatenate Strings(w4879, w4878, w4880) -> (w4877:string)
            n3946 = Concatenate Strings(w4869, w4870, w4868) -> (w4871:string)
            n3947 = Concatenate Strings(w4866, w4865, w4867) -> (w4864:string)
            n3948 = Concatenate Strings(w4863, w4875, w4892, w4833) -> (w4839:string)
            n3949 = Concatenate Strings(w4863, w4874, w4885, w4833) -> (w4838:string)
            n3950 = Concatenate Strings(w4863, w4873, w4884, w4833) -> (w4837:string)
            n3951 = Concatenate Strings(w4863, w4872, w4877, w4833) -> (w4836:string)
            n3952 = Concatenate Strings(w4863, w4862, w4871, w4833) -> (w4835:string)
            n3953 = Concatenate Strings(w4863, w4861, w4864, "\"}" ("string")) -> (w4834:string)
            n3954 = Concatenate Strings(w4840, w4839, w4838, w4837, w4836, w4835, w4834, "]}" ("string")) -> (w4831:string)
            n3955 = local read "SEN.RUN HRS"() -> (w4798:dbl)
            n3956 = disable-structure shown="Disabled" {
              frame Disabled {
                n3957 = local read "state"() -> (w4917:string[])
                n3958 = Delete From Array(array=w4917, index=0) -> (array with subset deleted=w4915:string[])  [unwired: 1 in, 1 out]
                n3959 = for {
                  N: 6 -> [_]
                  tunnel: w4915 -> [w4928] mode=indexing
                  tunnel: [w4927] -> w4914 mode=indexing
                  n3960 = Equal?(x=w4928, y="Warning") -> (x = y?=w4924:bool)
                  n3961 = Equal?(x=w4928, y="Healthy") -> (x = y?=w4921:bool)
                  n3962 = Select(t="2" ("y"), s=w4924, f="3" ("y")) -> (s? t:f=w4919:string)
                  n3963 = Select(t="1" ("y"), s=w4921, f=w4919) -> (s? t:f=w4927:string)
                }
                "state1" <- w4914
              }
              frame Enabled {
              }
            }
            n3964 = stacked-sequence {
              tunnel: w4831 -> [w4939 _ _]
              tunnel: [_ _ w4955] -> _
              frame #0 {
                (unwired) FALSE ("convert eol (F)")
                w4941 = enum16{"start", "end", "current"}."start" ("pos mode (0:2)")
                n3965 = local read "Path"() -> (w4935:path)
                n3966 = Path To String(path=w4935) -> (string=w4947:string)
                n3967 = Concatenate Strings(w4947, "\\", "Sensor File Name") -> (w4948:string)
                n3968 = local write "standard output 2"(" ") -> ()
                n3969 = String To Path(string=w4948) -> (path=w4938:path)
                n3970 = call <vilib>:"Open_Create_Replace File.vi"("advisory dialog? (display:T)"=FALSE, "function (open:0)"=T32."create or replace", "file path"=w4938) -> ("error out"=w4951:errorcluster, "refnum"=w4950:refnum<file>)  [unwired: 5 in, 2 out]
                n3971 = Set File Position(refnum=w4950, from (0:start)=w4941, error in=w4951) -> (refnum out=w4931:refnum<file>, error out=w4930:errorcluster)  [unwired: 1 in]
                n3972 = Write to Binary File(file (use dialog)=w4931, data=" ", error in=w4930, 5:FALSE ("prepend array or string size? (T)")) -> (refnum out=w4942:refnum<file>, error out=w4943:errorcluster)  [unwired: 2 in, 1 out]
                n3973 = Set File Position(offset (in bytes) (0)=w4941, refnum=w4942, error in=w4943) -> (refnum out=w4934:refnum<file>, error out=w4933:errorcluster)  [unwired: 1 in]
                n3974 = Write to Binary File(file (use dialog)=w4934, data=w4939, error in=w4933, 5:FALSE ("prepend array or string size? (T)")) -> (error out=w4937:errorcluster)  [unwired: 2 in, 2 out]
                n3975 = flat-sequence {
                  tunnel: w4938 -> [w4953]
                  tunnel: w4937 -> [_]
                  frame #0 {
                    n3976 = call <vilib>:"Read Characters From File.vi"("file path (dialog if empty)"=w4953) -> ("character string"=→"Sensor Health JSON string":string)  [unwired: 5 in, 3 out]
                  }
                }
                "SinglePoint  2" <- w4939
              }
              frame #1 {
              }
              frame #2 {
                (unwired) "\"Stored\": true" ("string")
                n3977 = call <vilib>:"System Exec.vi"("run minimized? (F)"=TRUE, "wait until completion? (T)"=TRUE, "working directory"=path "C:/LAB-IQ-NXT", "command line"="C:\\LAB-IQ-NXT\\JPostH.bat") -> ("standard error"=→"Respose From Server 2":string, "standard output"=w4958:string)  [unwired: 4 in, 2 out]
                "standard output 2" <- w4958
                n3978 = Match Pattern(string=w4958, regular expression="JSONH Check String") -> (match substring=w4956:string, offset past match=w4955:i32)  [unwired: 1 in, 2 out]
                n3979 = Equal?(x=w4956, y="JSONH Check String") -> (x = y?=→"Upload \nConfirmed 2":bool)
              }
            }
            n3980 = Divide(x=w4798, y=3600.0 ("f")) -> (x/y=w4791:dbl)
            n3981 = local read "run time"() -> (w4848:string[])
            n3982 = Round To Nearest(number=w4791) -> (nearest integer value=w4790:dbl)
            n3983 = Number To Decimal String(number=w4790) -> (decimal integer string=w4789:string)  [unwired: 1 in]
            n3984 = Index Array(array="Sensor Information", index (col) #1=0 ("disabled index (col)"), index (col) #2=1 ("index (col)"), index (col) #3=2 ("index (col)"), index (col) #4=3 ("index (col)")) -> (element #1=→"Sensor name":string[], element #2=→"model num":string[], element #3=→"run time":string[], element #4=→"state":string[])  [unwired: 4 in]
            n3985 = Insert Into Array(array=w4848, index=1, new element #1=w4789, new element #2=w4789, new element #3=w4789, new element #4=w4789, new element #5=w4789, new element #6=w4789) -> (w4813:string[])
            "run" <- w4813
            n3986 = local read "out"() -> (w4795:string[])
            n3987 = local read "Sensor Information"() -> (w4815:string[][])
            n3988 = Replace Array Subset(array=w4815, new element #1=w4813, index (col) #1=2 ("disabled index (col)"), new element #2=w4795, index (col) #2=3 ("index (col)")) -> (w4814:string[][])  [unwired: 2 in]
            n3989 = local write "Sensor Information"(w4814) -> ()
          }
        }
        n3990 = case shown="True" w4762 {
          frame False {
          }
          frame True {
            n3991 = Equal?(x="FLAG", y=0.0) -> (x = y?=w4779:bool)
            n3992 = case shown="False" w4779 {
              frame False {
                n3993 = Get Date/Time In Seconds() -> (seconds since 1Jan1904=w4785:timestamp)
                n3994 = local read "START 2"() -> (w4783:dbl)
                n3995 = To Double Precision Float(number=w4785) -> (double precision float=w4784:dbl)
                n3996 = Subtract(x=w4784, y=w4783) -> (x-y=→"SENSOR TIME  2":dbl)
              }
              frame True {
                n3997 = Get Date/Time In Seconds() -> (seconds since 1Jan1904=w4787:timestamp)
                n3998 = To Double Precision Float(number=w4787) -> (double precision float=→"START 2":dbl)
                n3999 = local write "FLAG"(100.0 ("FLAG")) -> ()
              }
            }
          }
        }
        n4000 = disable-structure shown="Disabled" {
          disable-tunnel: w4765 -> [w4774 _]
          disable-tunnel: [w4773 _] -> w4764
          frame Disabled {
            n4001 = local read "Json St Flg"() -> (w4772:bool)
            n4002 = case shown="True" w4772 {
              tunnel: w4774 -> [w4775 w4777]
              tunnel: [w4775 w4776] -> w4773
              frame False {
              }
